vi "state_machine.vi"() -> ()   [LabVIEW 2020]
uses:
  <vilib>/ErrorRing/Error Ring.xnode
panel:
  in  "Configuracion Alarma":dbl(slide) scale=0.0..100.0
  out "Tanques":dbl[](array[slide]) scale=0.0..100.0
  out "Alarmas":bool[](array[boolean])
  out "Estado actual":string
  in  "Direccion":path
  in  "stop":bool
  # "machine state"
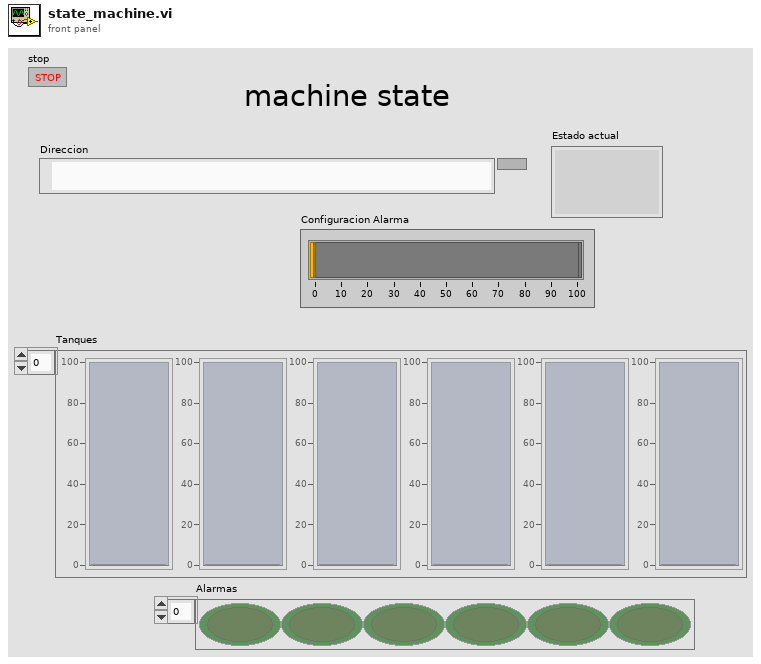
[diagram p1: front panel]
types:
  T1 = cluster{"Hardware":cluster{"Data Value":dbl[]}, "N values":cluster{"Cantidad":i32, "Lmax":dbl, "Lmin":dbl}, "alarmas":cluster{"warning":bool[]}, "Data Analisis":cluster{"Nombre Fichero":string, "formato":string, "Direccion":path, "refnum out":refnum<file>}}
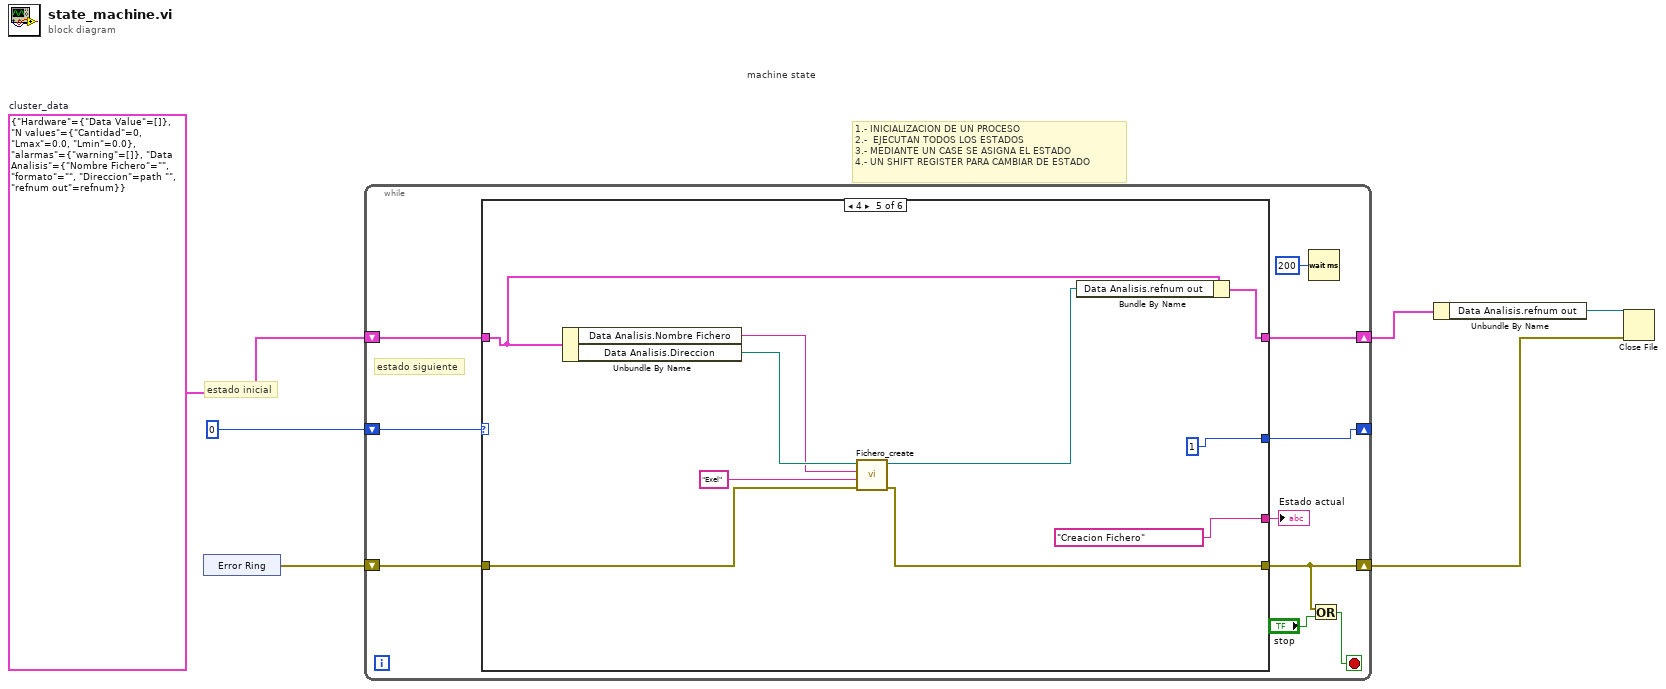
[diagram p0: block diagram]
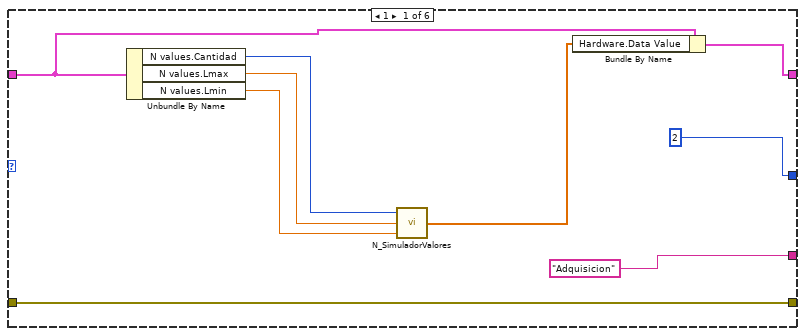
[diagram p2: hidden frame]
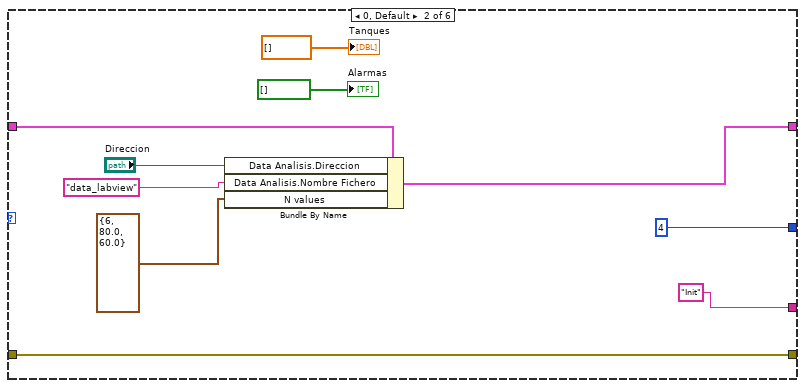
[diagram p3: hidden frame]
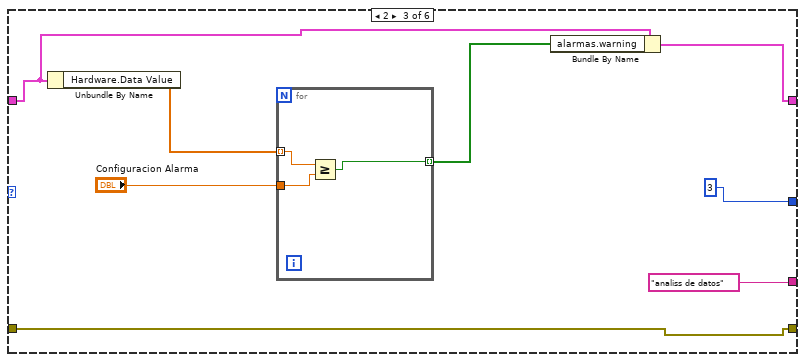
[diagram p4: hidden frame]
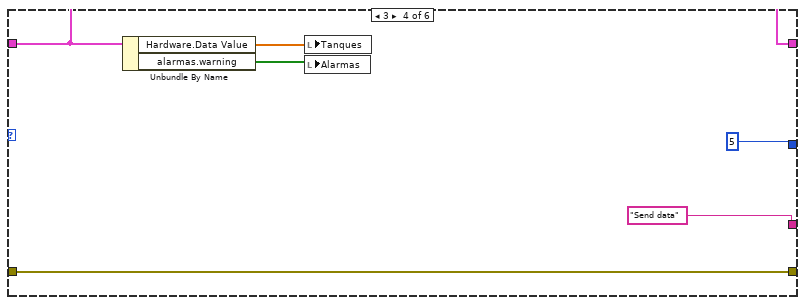
[diagram p5: hidden frame]
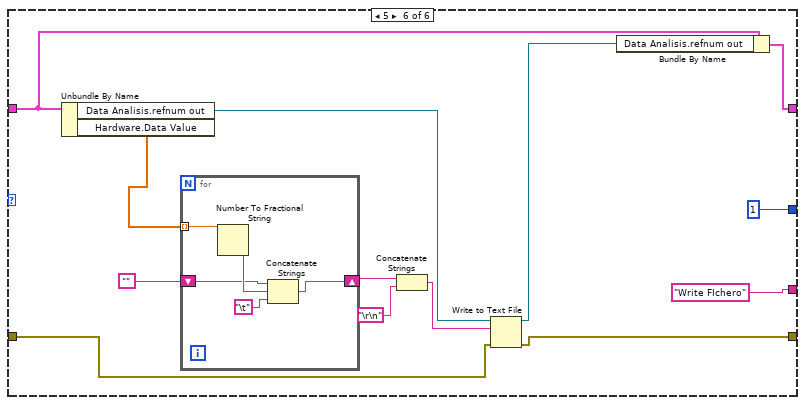
[diagram p6: hidden frame]
diagram:
  w5 = T1 {"Hardware"={"Data Value"=[]}, "N values"={"Cantidad"=0, "Lmax"=0.0, "Lmin"=0.0}, "alarmas"={"warning"=[]}, "Data Analisis"={"Nombre Fichero"="", "formato"="", "Direccion"=path "", "refnum out"=refnum}}  # cluster_data
  # "estado inicial"
  # "1.- INICIALIZACION DE UN PROCESO\n2.-  EJECUTAN TODOS LOS ESTADOS\n3.- MEDIANTE UN CASE SE ASIGNA EL ESTADO\n4.- UN SHIFT REGISTER PARA CAMBIAR DE ESTADO"
  # "machine state"
  n1 = xnode "Error Ring"() -> ("error out"=w4:errorcluster)
  n2 = while {
    shift-right: [w9] -> _
    shift-left: 0 -> [w16]
    shift-right: [w10] -> w3
    shift-left: w5 -> [w11]
    shift-right: [w13] -> w1
    shift-left: w4 -> [w15]
    stop <- w12 stop-if-true
    # "estado siguiente"
    n3 = case shown="4" w16 {
      tunnel: [w21 w35 w36 w49 w58 w68] -> w13
      tunnel: w15 -> [w21 w35 w36 w49 w59 w69]
      tunnel: w11 -> [w18 w34 w41 w50 w57 w66]
      tunnel: [w19 w33 w39 w50 w55 w65] -> w10
      tunnel: [2 4 3 5 1 1] -> w9
      tunnel: ["Adquisicion" "Init" "analiss de datos" "Send data" "Creacion Fichero" "Write FIchero"] -> w8
      frame 1 {
        n4 = Unbundle By Name(w18) -> ("N values.Cantidad"=w25:i32, "N values.Lmax"=w24:dbl, "N values.Lmin"=w23:dbl)
        n5 = call "N_SimuladorValores.vi"("Lim Max T"=w23, "Lim Min T"=w24, "Numeric"=w25) -> ("Array"=w17:dbl[])
        n6 = Bundle By Name(cluster=w18, "Hardware.Data Value"=w17) -> (w19:T1)
      }
      frame 0, Default {
        n7 = Bundle By Name(cluster=w34, "Data Analisis.Direccion"="Direccion", "Data Analisis.Nombre Fichero"="data_labview", "N values"=cluster{i32, dbl, dbl} {6, 80.0, 60.0}) -> (w33:T1)
        "Alarmas" <- bool[] []
        "Tanques" <- dbl[] []
      }
      frame 2 {
        n8 = Unbundle By Name(w41) -> ("Hardware.Data Value"=w43:dbl[])
        n9 = for {
          tunnel: w43 -> [w46] mode=indexing
          tunnel: "Configuracion Alarma" -> [w45]
          tunnel: [w44] -> w40 mode=indexing
          n10 = Greater Or Equal?(x=w46, y=w45) -> (x >= y?=w44:bool)
        }
        n11 = Bundle By Name(cluster=w41, "alarmas.warning"=w40) -> (w39:T1)
      }
      frame 3 {
        n12 = Unbundle By Name(w50) -> ("Hardware.Data Value"=w52:dbl[], "alarmas.warning"=w51:bool[])
        n13 = local write "Tanques"(w52) -> ()
        n14 = local write "Alarmas"(w51) -> ()
      }
      frame 4 {
        n15 = Unbundle By Name(w57) -> ("Data Analisis.Nombre Fichero"=w61:string, "Data Analisis.Direccion"=w62:path)
        n16 = call "Fichero_create.vi"("error in (no error)"=w59, "formato"="Exel", "Nombre Fichero"=w61, "Direccion"=w62) -> ("error out"=w58:errorcluster, "Byte Stream File out"=w56:refnum<file>)  [unwired: 6 in]
        n17 = Bundle By Name(cluster=w57, "Data Analisis.refnum out"=w56) -> (w55:T1)
      }
      frame 5 {
        n18 = Unbundle By Name(w66) -> ("Data Analisis.refnum out"=w71:refnum<file>, "Hardware.Data Value"=w75:dbl[])
        n19 = for {
          tunnel: w75 -> [w80] mode=indexing
          shift-right: [w76] -> w73
          shift-left: "" -> [w77]
          n20 = Number To Fractional String(number=w80) -> (F-format string=w79:string)  [unwired: 3 in]
          n21 = Concatenate Strings(w77, w79, "\t") -> (w76:string)
        }
        n22 = Concatenate Strings(w73, "\r\n") -> (w70:string)
        n23 = Write to Text File(file (use dialog)=w71, text=w70, error in=w69) -> (refnum out=w67:refnum<file>, error out=w68:errorcluster)  [unwired: 1 in, 1 out]
        n24 = Bundle By Name(cluster=w66, "Data Analisis.refnum out"=w67) -> (w65:T1)
      }
    }
    "Estado actual" <- w8
    n25 = Wait (ms)(milliseconds to wait=u32 200) -> ()  [unwired: 1 out]
    n26 = Or(x=w13, y="stop") -> (x .or. y?=w12:bool)
  }
  n27 = Unbundle By Name(w3) -> ("Data Analisis.refnum out"=w2:refnum<file>)
  n28 = Close File(refnum=w2, error in=w1) -> ()  [unwired: 2 out]
